vi "parseErrorCheck.vi"(2 "type":string, 3 "error in":errorcluster) -> (0 "error out":errorcluster)   [LabVIEW 2012]
doc: "Parses a message into an error check"
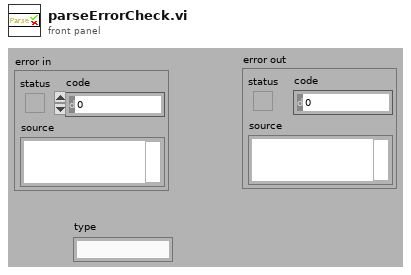
[diagram p1: front panel]
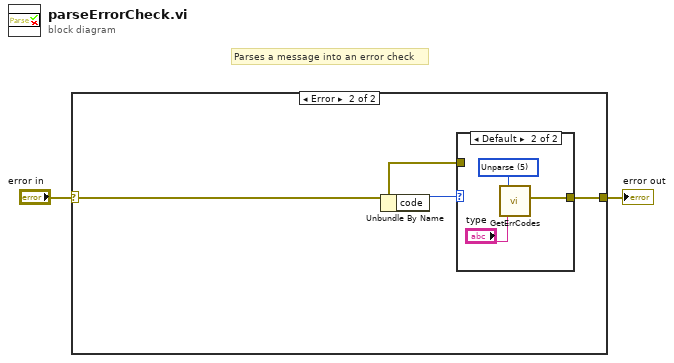
[diagram p0: block diagram]
diagram:
  # "Parses a message into an error check"
  n1 = case shown="Error" "error in" {
    selector: "error in" -> [w3 w4]
    tunnel: [w3 w6] -> w1
    frame No Error {
    }
    frame Error {
      n2 = Unbundle By Name(w4) -> ("code"=w5:i32)
      n3 = case shown="Default" w5 {
        tunnel: [w7 w9] -> w6
        tunnel: w4 -> [w7 _]
        frame 0 {
        }
        frame Default {
          w10 = u16 5 items=["TopicReadTimeout", "Read=SS", "GetQueueErr", "NoMaster", "Write=PS", "Unparse"] ("Error")
          n4 = call <userlib>:"GetErrCodes.vi"("Error"=w10, "Added Textt"="type") -> ("Error"=w9:errorcluster)  [unwired: 2 in]
        }
      }
    }
  }
  "error out" <- w1
